vi "order_centroid_MM.vi"(8 "update M":dbl[][](array[numeric]), 11 "parray":dbl[](array[numeric])) -> (0 "pmax_ind":i32, 1 "pmax":dbl, 2 "pmin_ind":i32, 3 "pmin":dbl, 4 "xmin":dbl[](array[numeric]), 5 "xmax":dbl[](array[numeric]), 6 "psmax":dbl, 7 "centroid":dbl[](array[numeric]))   [LabVIEW 2015]
panel:
  out "Sorted Indices":i32[](array[numeric])
  out "psmax_ind":i32
  out "xbar":dbl[](array[numeric])
  out "Sorted parray":dbl[](array[numeric])
  out "Sorted update M":dbl[][](array[numeric])
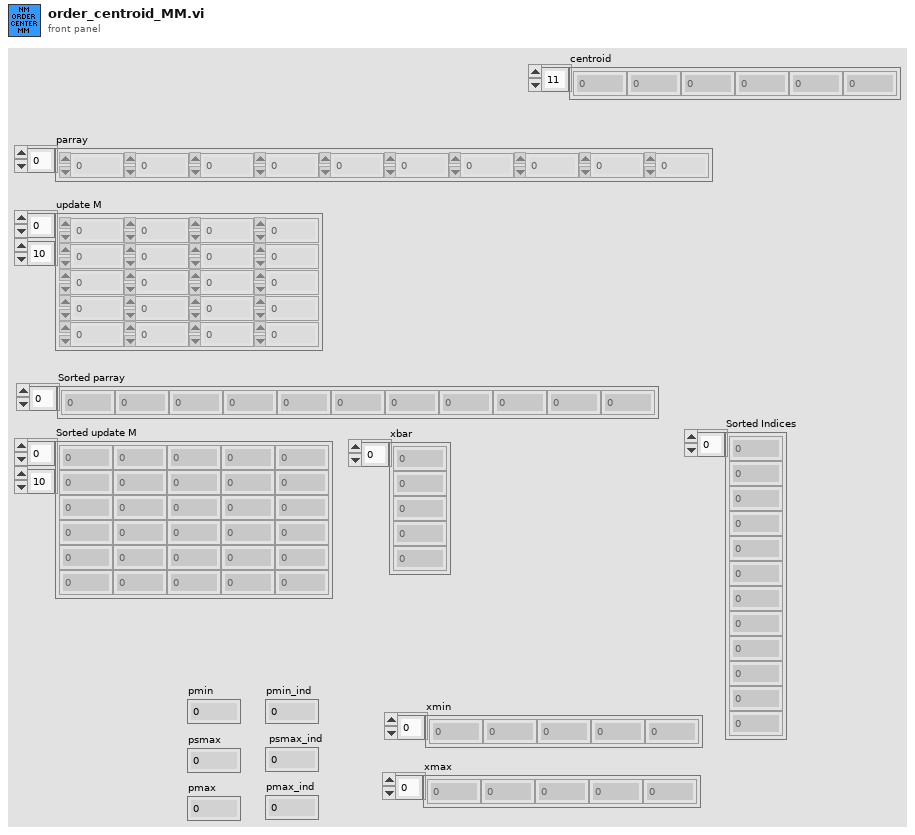
[diagram p1: front panel]
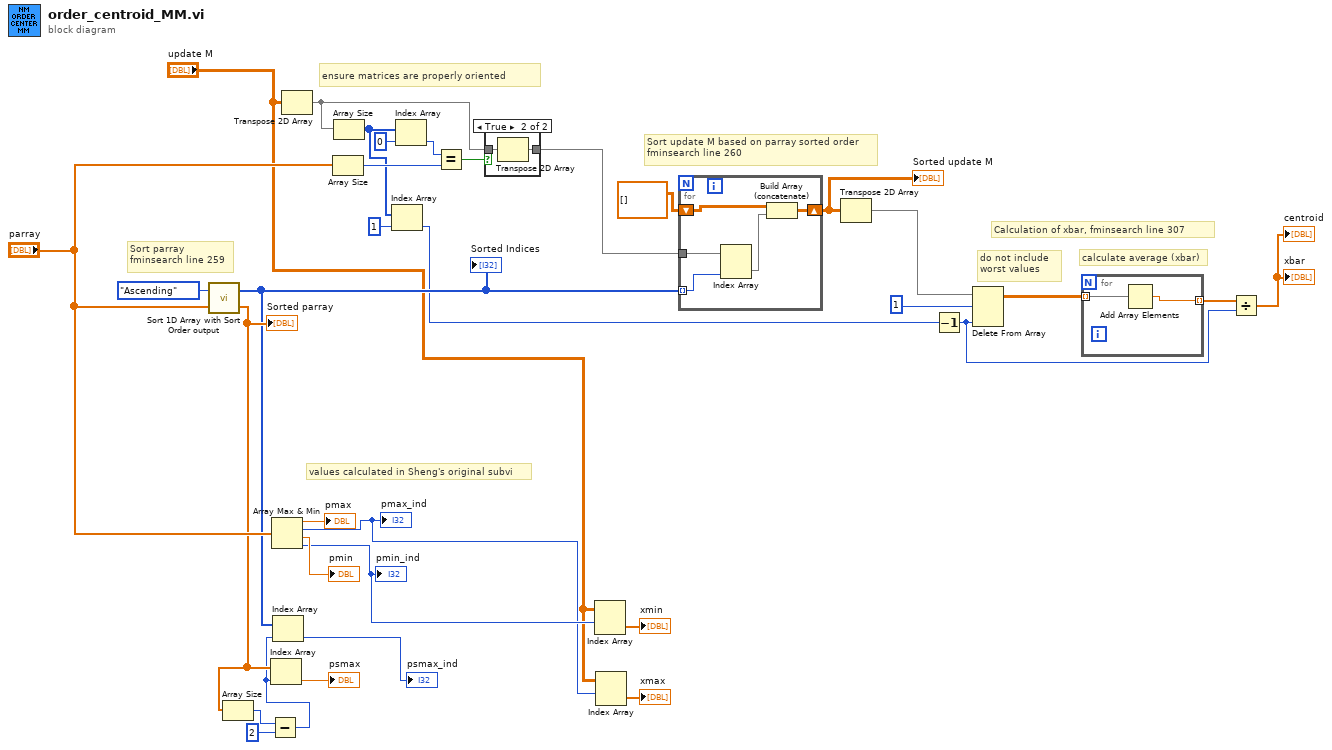
[diagram p0: block diagram]
diagram:
  # "values calculated in Sheng's original subvi"
  # "calculate average (xbar)"
  # "do not include \nworst values"
  # "Calculation of xbar, fminsearch line 307"
  # "ensure matrices are properly oriented"
  # "Sort update M based on parray sorted order\nfminsearch line 260"
  # "Sort parray \nfminsearch line 259"
  n1 = call "Sort 1D Array with Sort Order output.vi"("Disordered Array"="parray", "Sort Order"=enum16{"Ascending", "Descending"}."Ascending") -> ("Ordered Array"=w23:dbl[], "Original Indices"=w19:i32[])
  "Sorted parray" <- w23
  "Sorted Indices" <- w19
  n2 = Array Size(array=w23) -> (size(s)=w22:i32)
  n3 = Subtract(x=w22, y=2) -> (x-y=w18:i32)
  n4 = Index Array(array=w23, index=w18) -> (element=→"psmax":dbl)
  n5 = Array Max & Min(array="parray") -> (max value=→"pmax":dbl, max index (indices)=w13:i32, min value=→"pmin":dbl, min index (indices)=w15:i32)
  "pmin_ind" <- w15
  "pmax_ind" <- w13
  n6 = Index Array(array=w19, index=w18) -> (element=→"psmax_ind":i32)
  n7 = Transpose 2D Array(2D array="update M") -> (transposed array=w27:dbl[][])
  n8 = Array Size(array="parray") -> (size(s)=w32:i32)
  n9 = Array Size(array=w27) -> (size(s)=w3:i32[])
  n10 = Index Array(array=w3, index=1) -> (element=w2:i32)
  n11 = Index Array(array=w3, index=0) -> (element=w9:i32)
  n12 = Equal?(x=w9, y=w32) -> (x = y?=w30:bool)
  n13 = case shown="True" w30 {
    tunnel: w27 -> [w34 w36]
    tunnel: [w34 w35] -> w29
    frame False {
    }
    frame True {
      n14 = Transpose 2D Array(2D array=w36) -> (transposed array=w35:dbl[][])
    }
  }
  n15 = Index Array(array="update M", index (row)=w15) -> (element=→"xmin":dbl[])  [unwired: 1 in]
  n16 = Index Array(array="update M", index (row)=w13) -> (element=→"xmax":dbl[])  [unwired: 1 in]
  n17 = for {
    tunnel: w29 -> [w41]
    tunnel: w19 -> [w40] mode=indexing
    shift-right: [w38] -> w11
    shift-left: dbl[][] [] -> [w37]
    n18 = Index Array(array=w41, index (col)=w40) -> (element=w39:dbl[])  [unwired: 1 in]
    n19 = Build Array (concatenate)(w37, w39) -> (w38:dbl[][])
  }
  "Sorted update M" <- w11
  n20 = Transpose 2D Array(2D array=w11) -> (transposed array=w6:dbl[][])
  n21 = Decrement(x=w2) -> (x-1=w1:i32)
  n22 = Delete From Array(array=w6, length=1, index (col)=w1) -> (array with subset deleted=w7:dbl[][])  [unwired: 1 in, 1 out]
  n23 = for {
    tunnel: w7 -> [w43] mode=indexing
    tunnel: [w42] -> w10 mode=indexing
    n24 = Add Array Elements(numeric array=w43) -> (sum=w42:dbl)
  }
  n25 = Divide(x=w10, y=w1) -> (x/y=→"centroid" →"xbar":dbl[])
